vi "MenuHandler.vi"(5 "tree control":refnum<vi>, 6 "self reference":T1, 7 "main message queue":T2, 8 "error in":errorcluster, 9 "parameters":variant, 10 "menu string":string, 11 "CVT Engine Editor in":refnum<class "CVT Engine Editor.lvclass">) -> (0 "error out":errorcluster, 2 "Unhandled":bool, 3 "CVT Engine Editor out":refnum<class "CVT Engine Editor.lvclass">)   [LabVIEW 2013, in "CVT Engine Editor.lvclass"]
uses:
  CVT Engine Editor.lvclass
  <vilib>/NI/AMC/Message Queue.ctl
  <vilib>/NI/AMC/Message.ctl
  <vilib>/NI/Tools/Keyed Array/KeyedArray.ctl
  <vilib>/NI/Configuration Framework/Node/NodeRef.ctl
  <vilib>/NI/Configuration Framework/Node/NISE_CEF_Node.lvclass
  <vilib>/NI/Tag Bus Data Framework/Configuration Editor/Classes/Engine Parent/Engine Parent Editor Node.lvclass
  <vilib>/NI/Tools/Keyed Array/Tools_KeyedArray.lvlib
  <vilib>/NI/AMC/AMC.lvlib
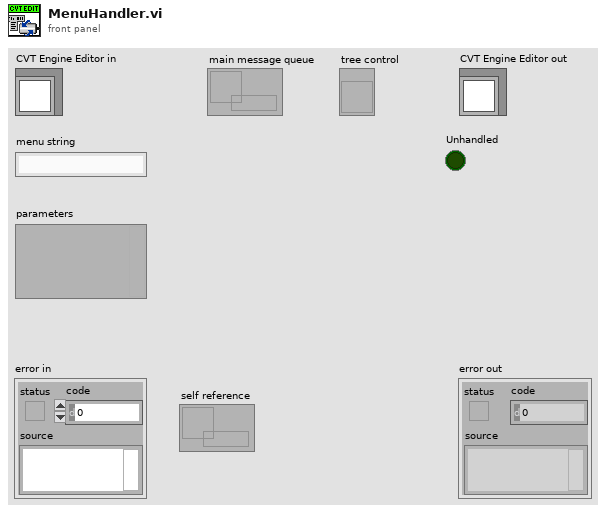
[diagram p1: front panel]
types:
  T1 = typedef "NISE_CEF_Node.lvclass/NodeRef.ctl" = refnum<data-value>
  T2 = typedef "AMC.lvlib/Message Queue.ctl" = refnum<queue>
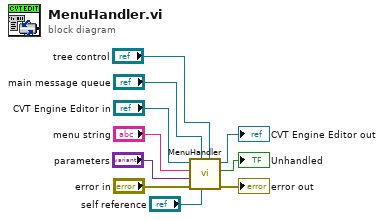
[diagram p0: block diagram]
diagram:
  n1 = call-parent "MenuHandler.vi"("tree control"="tree control", "self reference"="self reference", "main message queue"="main message queue", "error in"="error in", "parameters"="parameters", "menu string"="menu string", "NISE_CEF_serializable node in"="CVT Engine Editor in") -> ("error out"=→"error out":errorcluster, "Unhandled"=→"Unhandled":bool, "NISE_CEF_serializable node out"=→"CVT Engine Editor out":refnum<class "CVT Engine Editor.lvclass">)  [unwired: 2 in]
